vi "emi_Control enable and visibility single.vi"(0 "Control":refnum<vi>, 7 "State(Normal)":enum16{"Normal", "Disabled", "Grayed", "Hidden"}(ring), 11 "error in":errorcluster) -> (4 "Control out":refnum<vi>, 15 "error out":errorcluster)   [LabVIEW 2011]
doc: "Set state: Normal, Disabled, Grayed, hidden of array of controls.\n\nOn error: Does nothing."
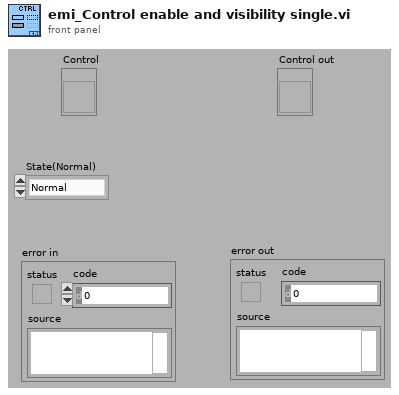
[diagram p1: front panel]
types:
  T1 = enum8{"Enabled", "Disabled", "Disabled and Grayed Out"}
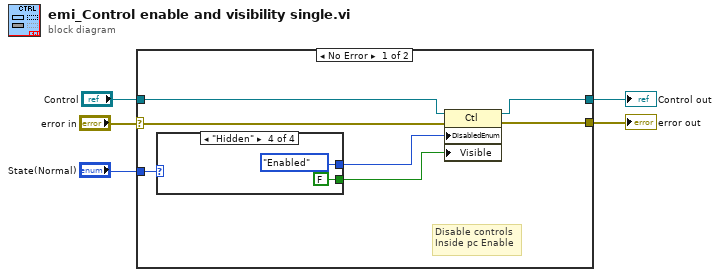
[diagram p0: block diagram]
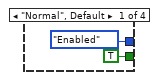
[diagram p2: hidden frame]
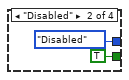
[diagram p3: hidden frame]
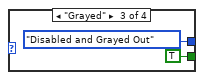
[diagram p4: hidden frame]
diagram:
  n1 = case shown="No Error" "error in" {
    selector: "error in" -> [w6 w22]
    tunnel: [w12 w21] -> w1
    tunnel: "Control" -> [w11 w21]
    tunnel: [w10 w22] -> w5
    tunnel: "State(Normal)" -> [w9 _]
    frame No Error {
      # "Disable controls\nInside pc Enable"
      n2 = case shown="\"Hidden\"" w9 {
        tunnel: [T1."Enabled" ("Disabled") T1."Disabled" ("Disabled") T1."Disabled and Grayed Out" ("Disabled") T1."Enabled" ("Disabled")] -> w8
        tunnel: [TRUE TRUE TRUE FALSE] -> w7
        frame "Normal", Default {
        }
        frame "Disabled" {
        }
        frame "Grayed" {
        }
        frame "Hidden" {
        }
      }
      n3 = property class="Ctl"(reference=w11, error in=w6, "DisabledEnum"=w8, "Visible"=w7) -> (reference out=w12:refnum<vi>, error out=w10:errorcluster)
    }
    frame Error {
    }
  }
  "error out" <- w5
  "Control out" <- w1
